vi "Spilit String.vi"(1 "Imput String":string="1TICA-2522") -> (0 "Output String":string)   [LabVIEW 2013]
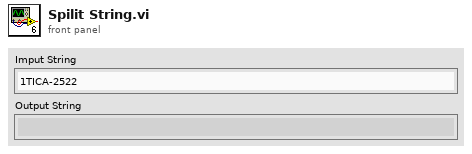
[diagram p1: front panel]
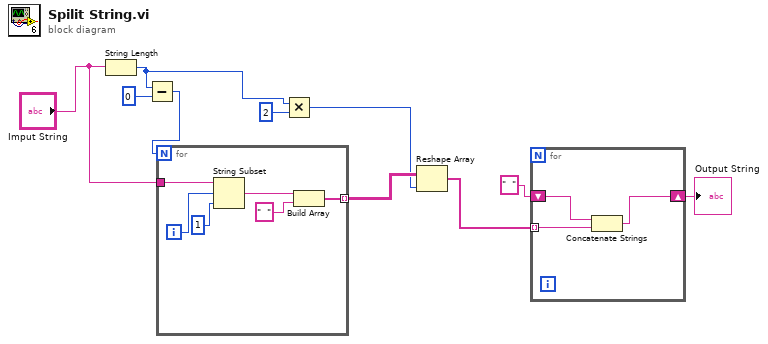
[diagram p0: block diagram]
diagram:
  n1 = String Length(string="Imput String") -> (length=w1:i32)
  n2 = Subtract(x=w1, y=0) -> (x-y=w5:i32)
  n3 = for {
    N: w5 -> [_]
    tunnel: "Imput String" -> [w16]
    tunnel: [w11] -> w8 mode=indexing
    i -> [w15]
    n4 = String Subset(string=w16, offset (0)=w15, length (rest)=1 ("length (rest)")) -> (substring=w13:string)
    n5 = Build Array(w13, "  " ("element")) -> (w11:string[])
  }
  n6 = Multiply(x=w1, y=2) -> (x*y=w6:i32)
  n7 = Reshape Array(w8, w6) -> (w3:string[])
  n8 = for {
    shift-right: [w19] -> w2
    shift-left: "  " ("element") -> [w18]
    tunnel: w3 -> [w17] mode=indexing
    n9 = Concatenate Strings(w18, w17) -> (w19:string)
  }
  "Output String" <- w2
